vi "Test Read Accelerometer.vi"() -> ()   [LabVIEW 2012]
panel:
  in  "Stop":bool
  in  "Rate":dbl=100.0
  out "Waveform Chart":dbl[][](graph)
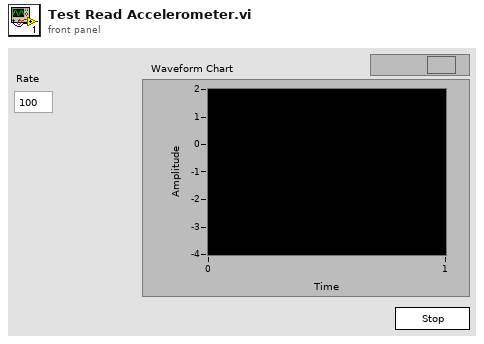
[diagram p1: front panel]
types:
  T1 = typedef "Accelerometer.ctl" = cluster{"Device":T2, "i2c configuration":T3}
  T2 = typedef "ni845xControl.ctl" = refnum<k21>
  T3 = typedef "ni845xI2cConfiguration.ctl" = refnum<k20>
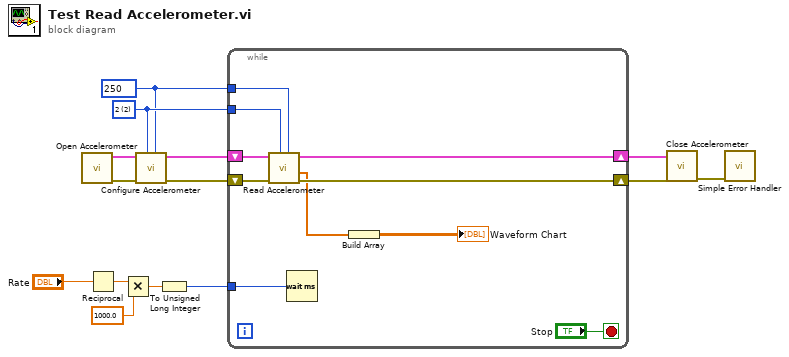
[diagram p0: block diagram]
diagram:
  w1 = u16 250 items=["250"=250, "500"=500, "1000"=1000, "2000"=2000] ("gyro range (deg/sec)")
  w2 = u16 2 items=["2"=2, "4"=4, "8"=8, "16"=16] ("accel range (g)")
  n1 = call "Open Accelerometer.vi"() -> ("error out"=w6:errorcluster, "Accelerometer"=w5:T1)  [unwired: 10 in]
  n2 = Reciprocal(x="Rate") -> (1/x=w13:dbl)
  n3 = Multiply(x=w13, y=1000.0) -> (x*y=w11:dbl)
  n4 = call "Configure Accelerometer.vi"("gyro range (deg/sec)"=w1, "accel range (g)"=w2, "error in (no error)"=w6, "Accelerometer"=w5) -> ("error out"=w3:errorcluster, "Accelerometer out"=w4:T1)  [unwired: 6 in]
  n5 = To Unsigned Long Integer(number=w11) -> (unsigned 32bit integer=w10:u32)
  n6 = while {
    shift-right: [w21] -> w9
    shift-left: w4 -> [w23]
    shift-right: [w20] -> w8
    shift-left: w3 -> [w22]
    tunnel: w10 -> [w19]
    tunnel: w2 -> [w18]
    tunnel: w1 -> [w17]
    stop <- "Stop" stop-if-true
    n7 = call "Read Accelerometer.vi"("gyro range (deg/sec)"=w17, "accel range (g)"=w18, "error in (no error)"=w22, "Accelerometer"=w23) -> ("error out"=w20:errorcluster, "gyro"=w15:dbl[], "Accelerometer out"=w21:T1)  [unwired: 3 in, 2 out]
    n8 = Wait (ms)(milliseconds to wait=w19) -> ()  [unwired: 1 out]
    n9 = Build Array(w15) -> (→"Waveform Chart":dbl[][])
  }
  n10 = call "Close Accelerometer.vi"("error in (no error)"=w8, "Accelerometer"=w9) -> ("error out"=w7:errorcluster)  [unwired: 9 in]
  n11 = call <vilib>:"Simple Error Handler.vi"("error in (no error)"=w7) -> ()  [unwired: 4 in, 5 out]
